vi "DAQEG_Get Waveform By Channel.vi"(8 "error in":errorcluster, 10 "DAQ Channel":string="Dev1/ai0") -> (0 "error out":errorcluster, 2 "waveform":waveform(dbl))   [LabVIEW 2016]
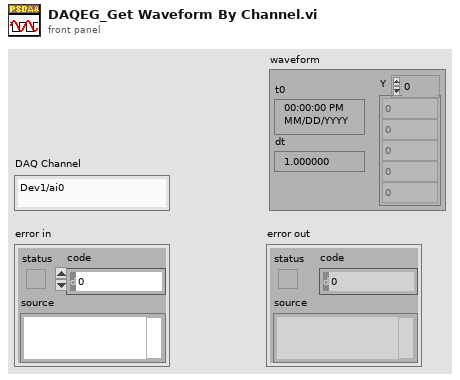
[diagram p1: front panel]
types:
  T1 = typedef "HardWare _ Data Queue Info.ctl" = cluster{"Q Name":string, "ch name[]":string[], "ch alias[]":string[]}
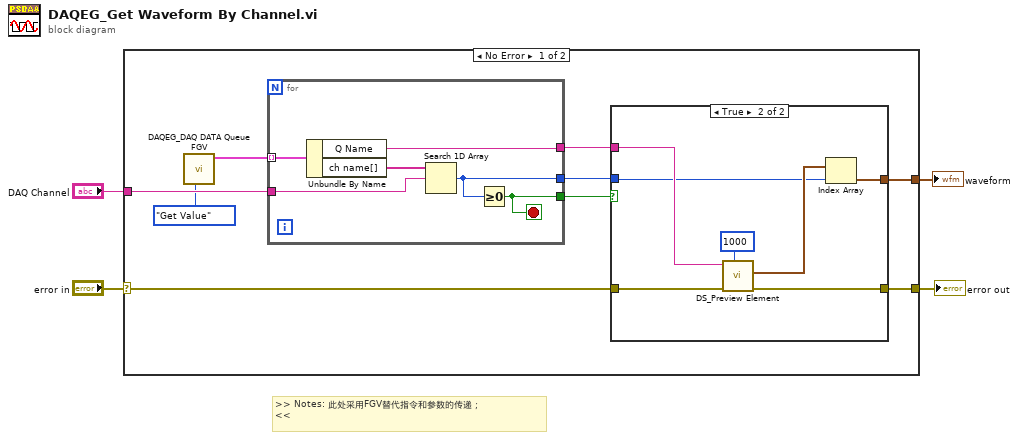
[diagram p0: block diagram]
diagram:
  # ">> Notes: 此处采用FGV替代指令和参数的传递；\n<<"
  n1 = case shown="No Error" "error in" {
    selector: "error in" -> [w5 w28]
    tunnel: "DAQ Channel" -> [w13 _]
    tunnel: [w12 w28] -> w3
    tunnel: [w8 _] -> w2
    frame No Error {
      n2 = call "DAQEG_DAQ DATA Queue FGV.vi"("Command"=enum16{"Initialize", "Get Value", "Set Value"}."Get Value") -> ("data queue[] out"=w6:T1[])  [unwired: 9 in, 1 out]
      n3 = for {
        tunnel: w6 -> [w27] mode=indexing
        tunnel: w13 -> [w25]
        tunnel: [w24] -> w11
        tunnel: [w23] -> w9
        tunnel: [w22] -> w10
        stop <- w22 stop-if-true
        n4 = Unbundle By Name(w27) -> ("Q Name"=w24:string, "ch name[]"=w26:string[])
        n5 = Search 1D Array(1D array=w26, element=w25) -> (index of element=w23:i32)  [unwired: 1 in]
        n6 = Greater Or Equal To 0?(x=w23) -> (x >= 0?=w22:bool)
      }
      n7 = case shown="True" w10 {
        tunnel: w5 -> [w14 w21]
        tunnel: [w14 w20] -> w12
        tunnel: w11 -> [_ w19]
        tunnel: w9 -> [_ w17]
        tunnel: [_ w16] -> w8
        frame False {
        }
        frame True {
          n8 = call "DS_Preview Element.vi"("Time Out(-1)"=1000, "error in"=w21, "Object Name"=w19) -> ("error out"=w20:errorcluster, "Wave"=w18:waveform(dbl)[])  [unwired: 6 in, 1 out]
          n9 = Index Array(array=w18, index=w17) -> (element=w16:waveform(dbl))
        }
      }
    }
    frame Error {
    }
  }
  "error out" <- w3
  "waveform" <- w2
